vi "Add Sink to Array.vi"(8 "error in (no error)":errorcluster, 10 "Sink":refnum<class "Sink.lvclass">, 11 "Registry in":refnum<class "Registry.lvclass">) -> (0 "error out":errorcluster, 3 "Registry out":refnum<class "Registry.lvclass">)   [LabVIEW 2020, in "LV Log.lvlib" / "Registry.lvclass"]
uses:
  Registry.lvclass
  Sink/Sink.lvclass
  Registry.lvclass/Registry.ctl
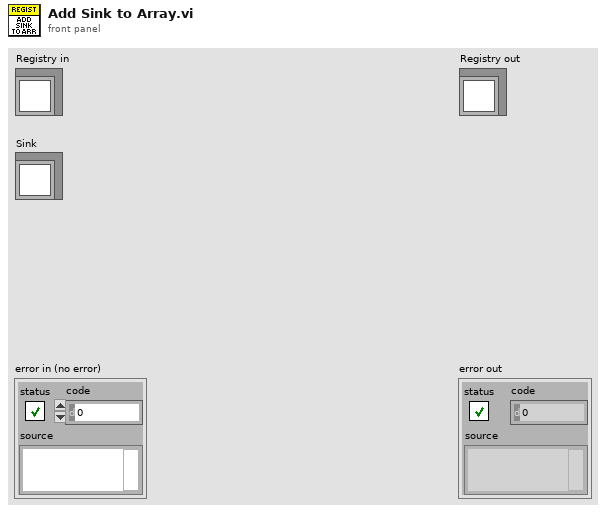
[diagram p1: front panel]
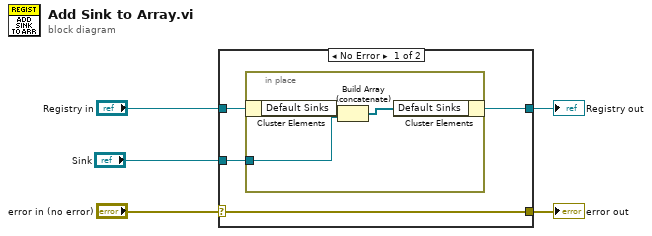
[diagram p0: block diagram]
diagram:
  n1 = case shown="No Error" "error in (no error)" {
    selector: "error in (no error)" -> [w9 w14]
    tunnel: [w9 w14] -> w4
    tunnel: [w7 w13] -> w2
    tunnel: "Registry in" -> [w8 w13]
    tunnel: "Sink" -> [w6 _]
    frame No Error {
      n2 = in-place {
        in-place-border: w6 -> [w10]
        n3 = in-place-cluster #1(w8) -> ("Default Sinks"=w12:refnum<class "Sink.lvclass">[])
        n4 = Build Array (concatenate)(w12, w10) -> (w11:refnum<class "Sink.lvclass">[])
        n5 = in-place-cluster #1("Default Sinks"=w11) -> (w7:refnum<class "Registry.lvclass">)
      }
    }
    frame Error {
    }
  }
  "error out" <- w4
  "Registry out" <- w2
